vi "Add Autosampler Step.vi"(8 "error in (no error)":errorcluster, 9 "Movie index":i32, 10 "Sweeps":T1[](array[typedef]), 11 "AutomationContext in":refnum<class "AutomationContext.lvclass">) -> (0 "error out":errorcluster, 3 "AutomationContext out":refnum<class "AutomationContext.lvclass">)   [LabVIEW 2023, in "Automation.lvlib" / "AutomationContext.lvclass"]
uses:
  AutomationContext.lvclass
  Resources/Type Defs/Param Sweep.ctl
  Resources/Type Defs/Sweep Parameter.ctl
  Resources/Type Defs/Camera Settings.ctl
  8a3729b4-80cc-4098-ac0d-2dcc27639522.vi
  87422d5c-a898-4e78-b7e3-b12e80407324.vi
  72709a6a-dc22-4607-b55f-041e86a4b367.vi
  91d38120-202a-4811-8d34-0beea14264ca.vi
  791957df-3dd3-4881-87fc-351f86b740d3.vi
  b0b38208-7a50-4606-a133-0504153f8b26.vi
  <vilib>/JDP Science/JSONtext/JSON text to Variant.vi
  <vilib>/JDP Science/JSONtext/LVClass Serializer/JSONtext LVClass Serializer.lvclass
  AutomationContext.lvclass/AutomationContext.ctl
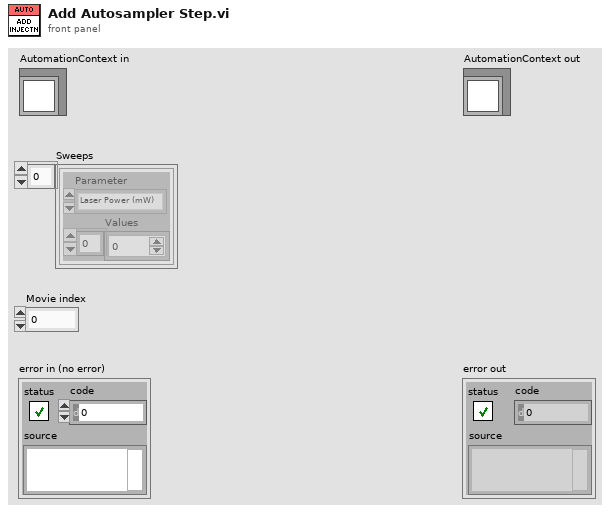
[diagram p1: front panel]
types:
  T1 = typedef "Param Sweep.ctl" = cluster{"Parameter":T2, "Values":dbl[]}
  T2 = typedef "Sweep Parameter.ctl" = enum16{"Laser Power (mW)", "Exposure Time (ms)", "Number of Frames", "Laser Line (1,2,3,4)", "Inject from Well"}
  T3 = cluster{"Area":enum16{"Home", "Well", "Wash Port"}, "Index":u16}
  T4 = typedef "Camera Settings.ctl" = cluster{"Exposure Time (ms)":dbl, "Binning":enum16{"1x1", "2x2", "4x4"}, "Scan Mode":i32, "Frames to Acquire":dbl, "Pixel Correction":bool, "Frames to Skip":u32, "File Path":path, "Duty cycle":dbl, "ALEX":bool, "Shutter Enable":bool[], "fluidics trigger, ms (0=disabled)":dbl, "Bit Depth":u16, "Image Width (px)":u16, "Image Height (px)":u16, "Horizontal Offset (px)":u16, "Vertical Offset (px)":u16}
  T5 = cluster{"Camera Settings":T4, "Injection Countdown":bool}
  T6 = cluster{"Tasks":cluster{"Action":enum16{"Next Field", "Next Lane", "Set Power", "Reset Power", "Autofocus", "Start Streaming", "Delay", "Finish Run", "Open Shutter", "Close Shutter", "AS Move To", "AS Set Fill Vol", "AS Set Valve", "AS Shake", "AS Wash Needle", "AS Lower Needle", "AS Raise Needle"}, "Parameters":string}[]}[]
  T7 = cluster{"Action":enum16{"Next Field", "Next Lane", "Set Power", "Reset Power", "Autofocus", "Start Streaming", "Delay", "Finish Run", "Open Shutter", "Close Shutter", "AS Move To", "AS Set Fill Vol", "AS Set Valve", "AS Shake", "AS Wash Needle", "AS Lower Needle", "AS Raise Needle"}, "Parameters":string}[]
  T8 = enum16{"Next Field", "Next Lane", "Set Power", "Reset Power", "Autofocus", "Start Streaming", "Delay", "Finish Run", "Open Shutter", "Close Shutter", "AS Move To", "AS Set Fill Vol", "AS Set Valve", "AS Shake", "AS Wash Needle", "AS Lower Needle", "AS Raise Needle"}
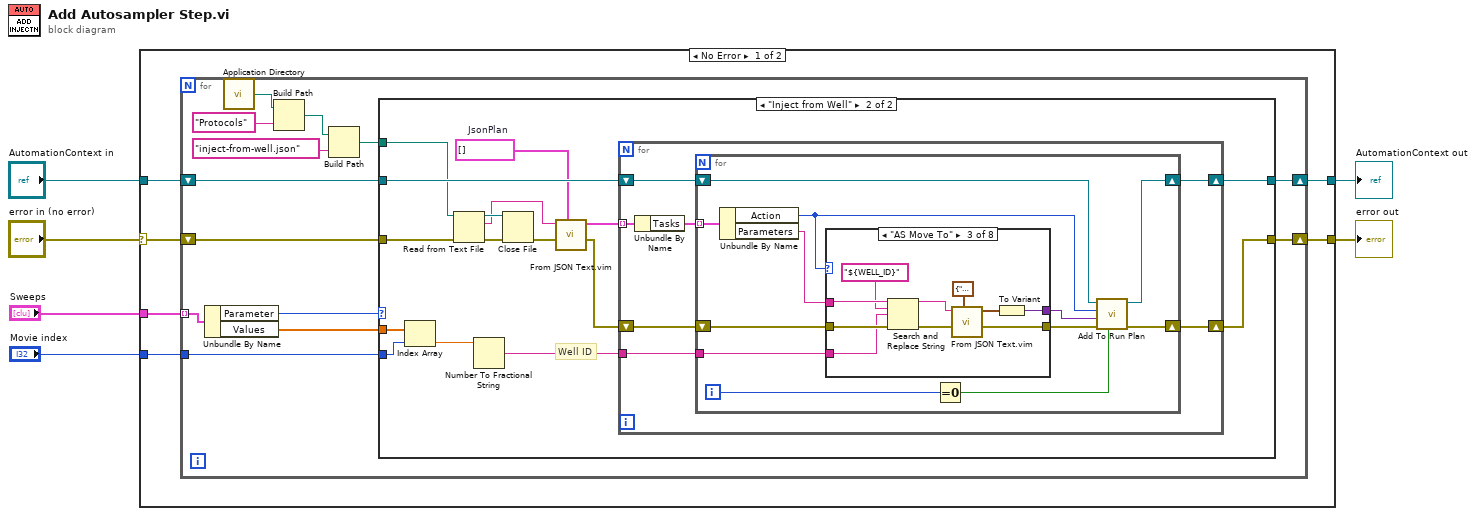
[diagram p0: block diagram]
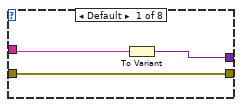
[diagram p3: hidden frame]
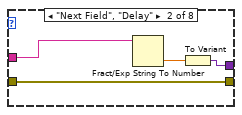
[diagram p4: hidden frame]
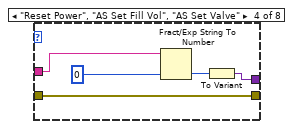
[diagram p5: hidden frame]
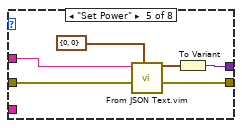
[diagram p6: hidden frame]
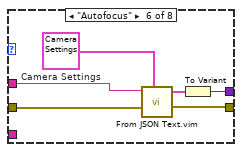
[diagram p7: hidden frame]
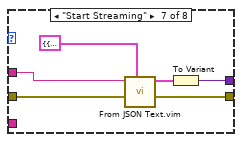
[diagram p8: hidden frame]
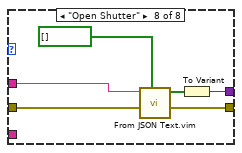
[diagram p9: hidden frame]
diagram:
  n1 = case shown="No Error" "error in (no error)" {
    selector: "error in (no error)" -> [w11 w110]
    tunnel: [w7 w110] -> w5
    tunnel: [w8 w109] -> w1
    tunnel: "AutomationContext in" -> [w10 w109]
    tunnel: "Sweeps" -> [w12 _]
    tunnel: "Movie index" -> [w9 _]
    frame No Error {
      n2 = for {
        tunnel: w12 -> [w25] mode=indexing
        tunnel: w9 -> [w19]
        shift-right: [w22] -> w8
        shift-left: w10 -> [w23]
        shift-right: [w20] -> w7
        shift-left: w11 -> [w21]
        n3 = Unbundle By Name(w25) -> ("Parameter"=w24:T2, "Values"=w18:dbl[])
        n4 = call <vilib>:"Application Directory.vi"() -> ("Application Directory"=w17:path)
        n5 = Build Path(base path=w17, name or relative path="Protocols") -> (appended path=w16:path)
        n6 = Build Path(base path=w16, name or relative path="inject-from-well.json") -> (appended path=w13:path)
        n7 = case shown="\"Inject from Well\"" w24 {
          tunnel: w23 -> [w27 w35]
          tunnel: [w27 w34] -> w22
          tunnel: w21 -> [w26 w41]
          tunnel: [w26 w36] -> w20
          tunnel: w19 -> [_ w42]
          tunnel: w18 -> [_ w43]
          tunnel: w13 -> [_ w28]
          frame Default {
          }
          frame "Inject from Well" {
            w33 = T6 []  # JsonPlan
            # "Well ID"
            n8 = Index Array(array=w43, index=w42) -> (element=w38:dbl)
            n9 = Read from Text File(file (use dialog)=w28, error in=w41) -> (refnum out=w30:refnum<file>, text=w29:string, error out=w32:errorcluster)  [unwired: 2 in, 1 out]
            n10 = Number To Fractional String(number=w38) -> (F-format string=w37:string)  [unwired: 3 in]
            n11 = Close File(refnum=w30, error in=w32) -> (error out=w31:errorcluster)  [unwired: 1 out]
            n12 = call "From JSON Text.vim"("Data Type and Default Value"=w33, "error in (no error)"=w31, "JSON"=w29) -> ("error out"=w39:errorcluster, "Data out"=w40:T6)  [unwired: 7 in]
            n13 = for "For Loop over parallel blocks" {
              tunnel: w40 -> [w50] mode=indexing
              shift-right: [w48] -> w36
              shift-left: w39 -> [w47]
              tunnel: w37 -> [w46]
              shift-right: [w44] -> w34
              shift-left: w35 -> [w45]
              n14 = Unbundle By Name(w50) -> ("Tasks"=w49:T7)
              n15 = for {
                tunnel: w49 -> [w62] mode=indexing
                shift-right: [w57] -> w48
                shift-left: w47 -> [w60]
                tunnel: w46 -> [w59]
                shift-right: [w55] -> w44
                shift-left: w45 -> [w56]
                i -> [w52]
                n16 = Unbundle By Name(w62) -> ("Action"=w53:T8, "Parameters"=w61:string)
                n17 = case shown="\"AS Move To\"" w53 {
                  tunnel: w61 -> [w65 w69 w74 w82 w87 w95 w97 w104]
                  tunnel: [w64 w68 w76 w80 w85 w92 w99 w105] -> w54
                  tunnel: w60 -> [w63 w66 w75 w84 w90 w96 w101 w108]
                  tunnel: [w63 w66 w79 w84 w89 w94 w100 w107] -> w58
                  tunnel: w59 -> [_ _ w70 _ _ _ _ _]
                  frame Default {
                    n18 = To Variant(anything=w65) -> (Variant=w64:variant)
                  }
                  frame "Next Field", "Delay" {
                    n19 = Fract/Exp String To Number(string=w69) -> (number=w67:dbl)  [unwired: 3 in, 1 out]
                    n20 = To Variant(anything=w67) -> (Variant=w68:variant)
                  }
                  frame "AS Move To" {
                    n21 = Search and Replace String(input string=w74, search string="${WELL_ID}", replace string=w70, error in=w75) -> (result string=w72:string, error out=w73:errorcluster)  [unwired: 4 in, 2 out]
                    n22 = call "From JSON Text.vim"("Data Type and Default Value"=T3 {"Area"=enum."Home", "Index"=0}, "error in (no error)"=w73, "JSON"=w72) -> ("error out"=w79:errorcluster, "Data out"=w77:T3)  [unwired: 7 in]
                    n23 = To Variant(anything=w77) -> (Variant=w76:variant)
                  }
                  frame "Reset Power", "AS Set Fill Vol", "AS Set Valve" {
                    n24 = Fract/Exp String To Number(string=w82, default (0 dbl)=u16 0 ("Volume, uL")) -> (number=w83:u16)  [unwired: 2 in, 1 out]
                    n25 = To Variant(anything=w83) -> (Variant=w80:variant)
                  }
                  frame "Set Power" {
                    n26 = call "From JSON Text.vim"("Data Type and Default Value"=cluster{i32, "Laser Power (mW)":u32} {0, "Laser Power (mW)"=0} ("output cluster"), "error in (no error)"=w90, "JSON"=w87) -> ("error out"=w89:errorcluster, "Data out"=w86:cluster{i32, "Laser Power (mW)":u32})  [unwired: 7 in]
                    n27 = To Variant(anything=w86) -> (Variant=w85:variant)
                  }
                  frame "Autofocus" {
                    w91 = T4 {"Exposure Time (ms)"=100.0, "Binning"=enum."2x2", "Scan Mode"=0, "Frames to Acquire"=1000.0, "Pixel Correction"=TRUE, "Frames to Skip"=0, "File Path"=path "", "Duty cycle"=0.2, "ALEX"=FALSE, "Shutter Enable"=[], "fluidics trigger, ms (0=disabled)"=0.0, "Bit Depth"=0, "Image Width (px)"=0, "Image Height (px)"=0, "Horizontal Offset (px)"=0, "Vertical Offset (px)"=0}  # Camera Settings
                    n28 = call "From JSON Text.vim"("Data Type and Default Value"=w91, "error in (no error)"=w96, "JSON"=w95) -> ("error out"=w94:errorcluster, "Data out"=w93:T4)  [unwired: 7 in]
                    n29 = To Variant(anything=w93) -> (Variant=w92:variant)
                  }
                  frame "Start Streaming" {
                    n30 = call "From JSON Text.vim"("Data Type and Default Value"=T5 {"Camera Settings"={"Exposure Time (ms)"=0.0, "Binning"=enum."1x1", "Scan Mode"=0, "Frames to Acquire"=0.0, "Pixel Correction"=FALSE, "Frames to Skip"=0, "File Path"=path "", "Duty cycle"=0.0, "ALEX"=FALSE, "Shutter Enable"=[], "fluidics trigger, ms (0=disabled)"=0.0, "Bit Depth"=0, "Image Width (px)"=0, "Image Height (px)"=0, "Horizontal Offset (px)"=0, "Vertical Offset (px)"=0}, "Injection Countdown"=FALSE} ("cluster"), "error in (no error)"=w101, "JSON"=w97) -> ("error out"=w100:errorcluster, "Data out"=w102:T5)  [unwired: 7 in]
                    n31 = To Variant(anything=w102) -> (Variant=w99:variant)
                  }
                  frame "Open Shutter" {
                    n32 = call "From JSON Text.vim"("Data Type and Default Value"=bool[] [] ("Array"), "error in (no error)"=w108, "JSON"=w104) -> ("error out"=w107:errorcluster, "Data out"=w106:bool[])  [unwired: 7 in]
                    n33 = To Variant(anything=w106) -> (Variant=w105:variant)
                  }
                }
                n34 = Equal To 0?(x=w52) -> (x = 0?=w51:bool)
                n35 = call "Add To Run Plan.vi"("New parallel block?"=w51, "error in (no error)"=w58, "Parameters"=w54, "Action"=w53, "AutomationContext in"=w56) -> ("error out"=w57:errorcluster, "AutomationContext out"=w55:refnum<class "AutomationContext.lvclass">)  [unwired: 5 in]
              }
            }
          }
        }
      }
    }
    frame Error {
    }
  }
  "error out" <- w5
  "AutomationContext out" <- w1
